vi "Experiment header-STATS section logic.vi"(11 "Logging queue element":T1 {"Frame Size" items=["100X100"=100, "128X128"=128, "200X200"=200, "256X256"=256, "512X512"=512, "1024x1024"=1024, "2048x2048"=2048]; "Dwell time (us)" format="%#.6g"}) -> (0 "error out":errorcluster)   [LabVIEW 2017]
uses:
  Typedefs/Logging queue element.ctl
  Typedefs/Imaging Protocols enum.ctl
  Typedefs/Frame Size.ctl
  Typedefs/Acquired points count.ctl
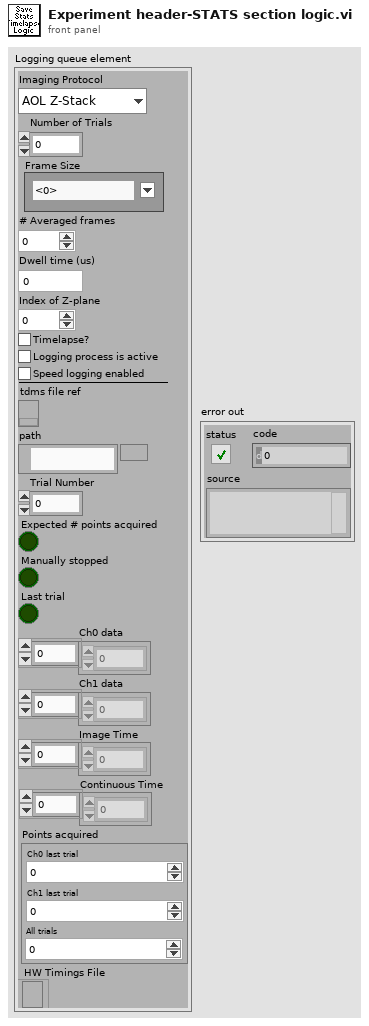
[diagram p1: front panel]
types:
  T1 = typedef "Logging queue element.ctl" = cluster{"Imaging Protocol":T2, "Number of Trials":u16, "Frame Size":T3, "# Averaged frames":u16, "Dwell time (us)":dbl, "Index of Z-plane":i32, "Timelapse?":bool, "Logging process is active":bool, "Speed logging enabled":bool, "tdms file ref":refnum<k34>, "path":path, "Trial Number":i32, "Expected # points acquired":bool, "Manually stopped":bool, "Last trial":bool, "Ch0 data":u32[], "Ch1 data":u32[], "Image Time":u64[], "Continuous Time":u64[], "Points acquired":T4, "HW Timings File":refnum<file>}
  T2 = typedef "Imaging Protocols enum.ctl" = enum16{"AOL Z-Stack", "Motor Z Stack", "Functional Acquisition", "Single Plane Acquisition", "Volume Acquisition", "Live Imaging", "Live Plane Imaging", "Live Volume Imaging"}
  T3 = typedef "Frame Size.ctl" = u16
  T4 = typedef "Acquired points count.ctl" = cluster{"Ch0 last trial":u64, "Ch1 last trial":u64, "All trials":u64}
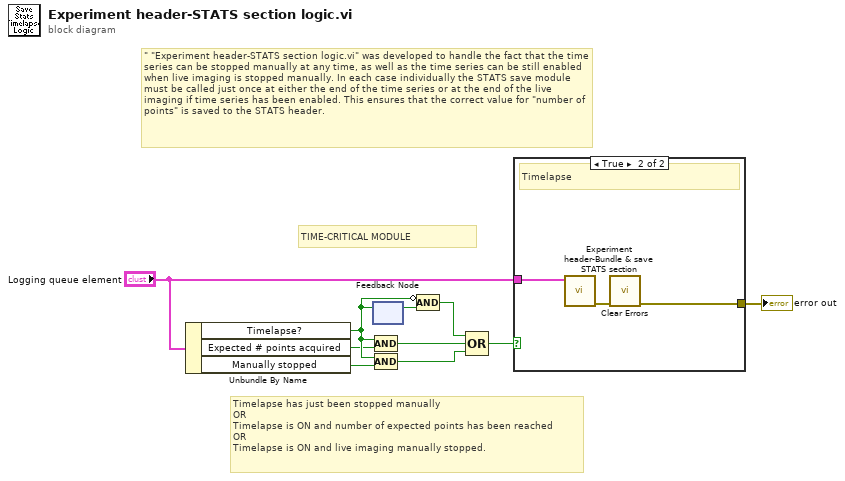
[diagram p0: block diagram]
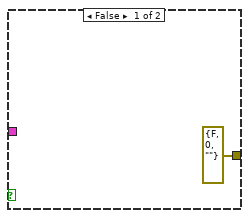
[diagram p2: hidden frame]
diagram:
  # "TIME-CRITICAL MODULE"
  # "Timelapse has just been stopped manually\nOR\nTimelapse is ON and number of expected points has been reached\nOR\nTimelapse is ON and live imaging manually stopped."
  # "\"\t\"Experiment header-STATS section logic.vi\" was developed to handle the fact that the time series can be stopped manually at any time, as well as the time series can be still enabled when live imaging is stopped manually. In each case individually the STATS save module must be called just once at either the end of the time series or at the end of the live imaging if time series has been enabled. This ensures that the correct value for \"number of points\" is saved to the STATS header."
  n1 = Unbundle By Name("Logging queue element") -> ("Timelapse?"=w8:bool, "Expected # points acquired"=w6:bool, "Manually stopped"=w9:bool)
  n2 = feedback #1() -> (w3:bool)  [unwired: 1 in]
  n3 = feedback-in #1(w8) -> ()
  n4 = Compound Arithmetic op=AND(w8, w6) -> (w7:bool)
  n5 = Compound Arithmetic op=AND(w8, w9) -> (w10:bool)
  n6 = Compound Arithmetic op=AND(invert w8, w3) -> (w5:bool)
  n7 = Compound Arithmetic op=OR(w5, w7, w10) -> (w4:bool)
  n8 = case shown="True" w4 {
    tunnel: "Logging queue element" -> [_ w14]
    tunnel: [errorcluster {"status"=FALSE, "code"=0, "source"=""} ("error out") w12] -> w1
    frame False {
    }
    frame True {
      # "Timelapse"
      n9 = call "Experiment header-Bundle & save STATS section.vi"("Logging queue element"=w14) -> ("error out"=w13:errorcluster)  [unwired: 10 in]
      n10 = call <vilib>:"Clear Errors.vi"("error in (no error)"=w13) -> ("error out"=w12:errorcluster)  [unwired: 5 in, 1 out]
    }
  }
  "error out" <- w1
